vi "Cockpit UDP Sender IRISSv2.vi"(6 "actual_gripper":sgl, 8 "actual_rotation":sgl, 9 "actual_Z":sgl, 10 "actual_Y":sgl, 11 "actual_X":sgl) -> ()   [LabVIEW 2016]
panel:
  in  "stop 2":bool
  in  "actual_X 2":sgl
  in  "actual_Y 2":sgl
  in  "actual_Z 2":sgl
  in  "actual_rotation 2":sgl
  in  "actual_gripper 2":sgl
  in  "actual_tool_insertion 2":sgl
  in  "tool_retina_distance 2":sgl
  in  "tool_retina_distance":sgl
  in  "actual_tool_insertion":sgl
  in  "stop":bool
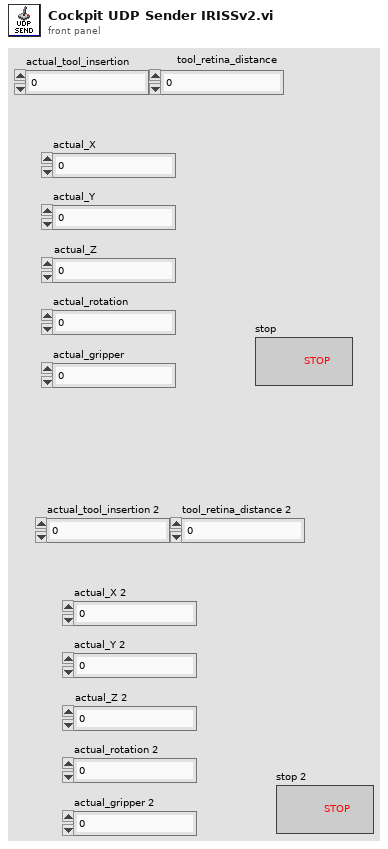
[diagram p1: front panel]
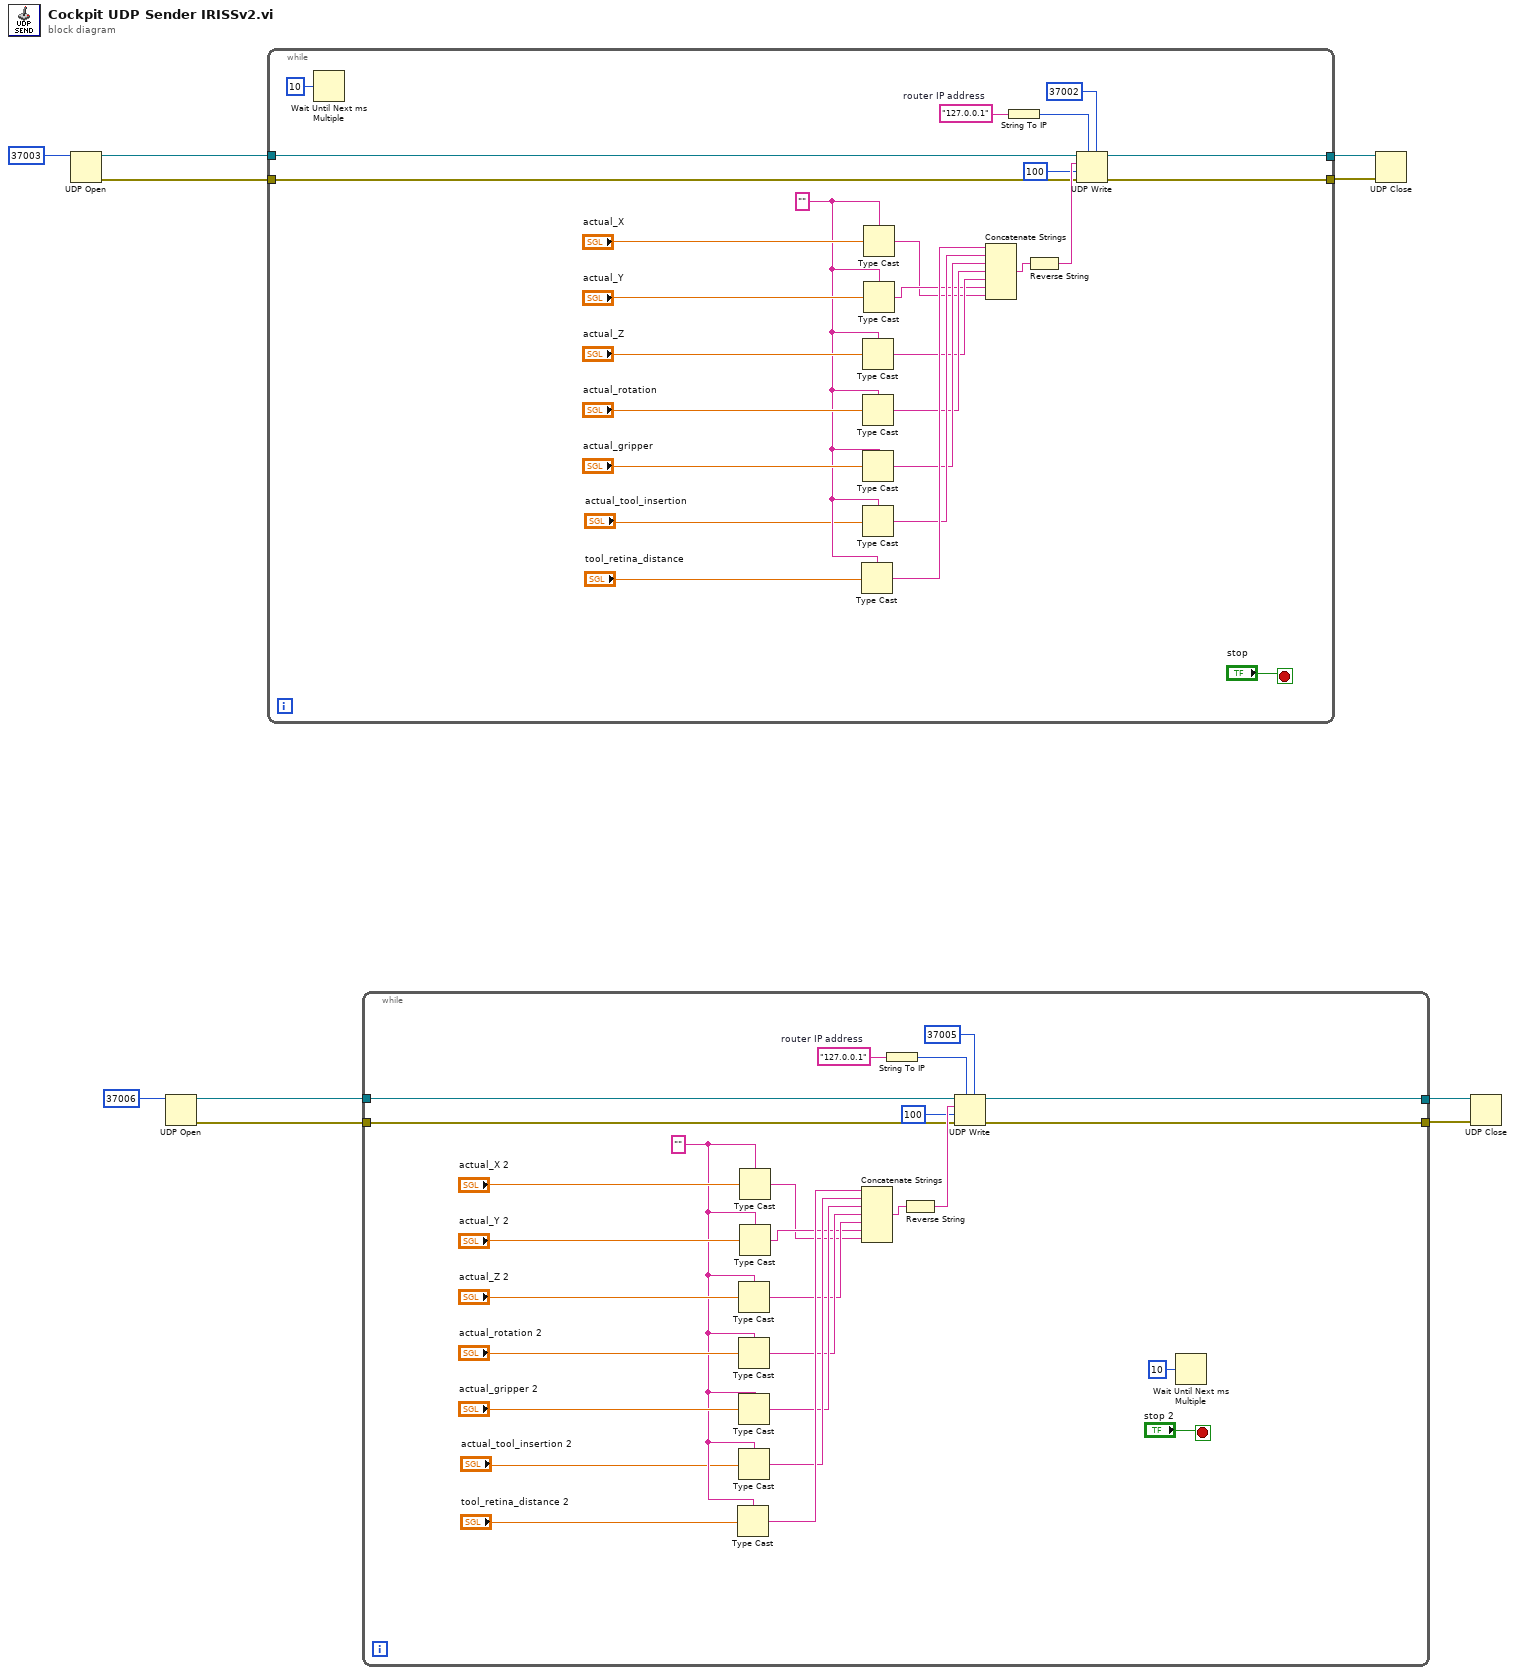
[diagram p0: block diagram]
diagram:
  n1 = UDP Open(11:u16 37003 ("port")) -> (port=w9:refnum<k16>, 0:w7:errorcluster)  [unwired: 4 in, 1 out]
  n2 = UDP Open(11:u16 37006 ("port")) -> (port=w4:refnum<k16>, 0:w2:errorcluster)  [unwired: 4 in, 1 out]
  n3 = while {
    tunnel: w9 -> [w31]
    tunnel: [w36] -> w8
    tunnel: w7 -> [w30]
    tunnel: [w35] -> w6
    stop <- "stop" stop-if-true
    w15 = "127.0.0.1"  # router IP address
    w24 = "" ("reversed")
    n4 = Wait Until Next ms Multiple(millisecond multiple=u32 10) -> ()  [unwired: 1 out]
    n5 = Type Cast(type=w24, x="tool_retina_distance") -> (*(type *) &x=w23:string)
    n6 = Type Cast(type=w24, x="actual_Z") -> (*(type *) &x=w19:string)
    n7 = Type Cast(type=w24, x="actual_rotation") -> (*(type *) &x=w20:string)
    n8 = Type Cast(type=w24, x="actual_gripper") -> (*(type *) &x=w21:string)
    n9 = Type Cast(type=w24, x="actual_tool_insertion") -> (*(type *) &x=w22:string)
    n10 = Type Cast(type=w24, x="actual_X") -> (*(type *) &x=w17:string)
    n11 = Type Cast(type=w24, x="actual_Y") -> (*(type *) &x=w18:string)
    n12 = Concatenate Strings(w23, w22, w21, w20, w19, w18, w17) -> (w34:string)
    n13 = String To IP(1:w15) -> (0:w14:u32)
    n14 = Reverse String(1:w34) -> (0:w33:string)
    n15 = UDP Write(address=w14, port or service name=u16 37002, connection ID=w31, data in=w33, 8:w30, 9:100 ("timeout ms (25000)")) -> (error out=w35:errorcluster, 3:w36:refnum<k16>)
  }
  n16 = while {
    tunnel: w4 -> [w58]
    tunnel: [w63] -> w3
    tunnel: w2 -> [w57]
    tunnel: [w62] -> w1
    stop <- "stop 2" stop-if-true
    w42 = "127.0.0.1"  # router IP address
    w51 = "" ("reversed")
    n17 = Type Cast(type=w51, x="tool_retina_distance 2") -> (*(type *) &x=w50:string)
    n18 = Type Cast(type=w51, x="actual_Z 2") -> (*(type *) &x=w46:string)
    n19 = Type Cast(type=w51, x="actual_rotation 2") -> (*(type *) &x=w47:string)
    n20 = Type Cast(type=w51, x="actual_gripper 2") -> (*(type *) &x=w48:string)
    n21 = Type Cast(type=w51, x="actual_tool_insertion 2") -> (*(type *) &x=w49:string)
    n22 = Type Cast(type=w51, x="actual_X 2") -> (*(type *) &x=w44:string)
    n23 = Type Cast(type=w51, x="actual_Y 2") -> (*(type *) &x=w45:string)
    n24 = Concatenate Strings(w50, w49, w48, w47, w46, w45, w44) -> (w61:string)
    n25 = String To IP(1:w42) -> (0:w41:u32)
    n26 = Reverse String(1:w61) -> (0:w60:string)
    n27 = UDP Write(address=w41, port or service name=u16 37005, connection ID=w58, data in=w60, 8:w57, 9:100 ("timeout ms (25000)")) -> (error out=w62:errorcluster, 3:w63:refnum<k16>)
    n28 = Wait Until Next ms Multiple(millisecond multiple=u32 10) -> ()  [unwired: 1 out]
  }
  n29 = UDP Close(connection ID=w8, 8:w6) -> ()  [unwired: 2 out]
  n30 = UDP Close(connection ID=w3, 8:w1) -> ()  [unwired: 2 out]
